vi "Test Get All Items.vi"(8 "error in (no error)":errorcluster, 11 "Result Model Result Recording Test in":refnum<class "Result Model Result Recording Test.lvclass">) -> (0 "error out":errorcluster, 3 "Result Model Result Recording Test out":refnum<class "Result Model Result Recording Test.lvclass">)   [LabVIEW 2020, in "Result Model Result Recording Test.lvclass"]
uses:
  Result Model Result Recording Test.lvclass
  Result Model Result Recording Test.lvclass/Result Model Result Recording Test.ctl
  Result Model/Result Model.lvclass
  Result/Type.ctl
  Result/Result.lvlib
  Result/Status.ctl
  Result/Result.ctl
  ae2c71b8-32bb-49d1-8500-0119bfec74ff.vi
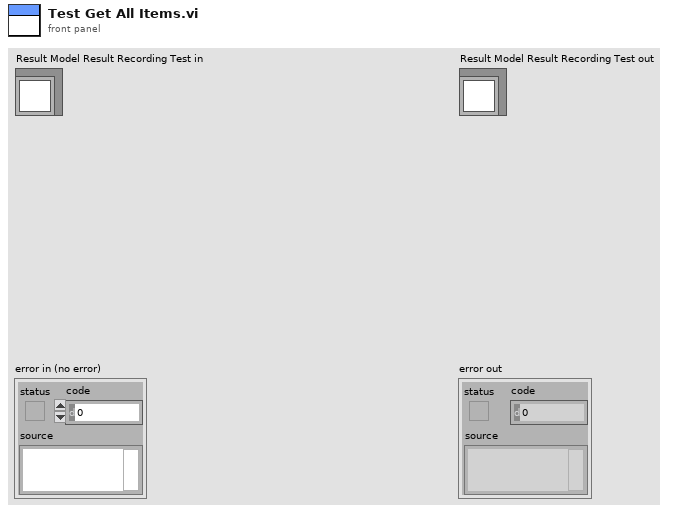
[diagram p1: front panel]
types:
  T1 = typedef "Result.lvlib/Result.ctl" = cluster{"Name":string, "Message":string, "Description":string, "Status":T2, "Result Type":T3, "Execution Time":dbl}
  T2 = typedef "Result.lvlib/Status.ctl" = enum16{"", "Passed", "Failed", "Error", "Skipped", "Setup Error", "Broken", "Teardown Error"}
  T3 = typedef "Result.lvlib/Type.ctl" = enum16{"Method", "Case", "Suite", "Pass", "Fail", "Skip", "Pass if", "Fail if", "Pass if Error", "Fail if Error", "Pass if Equal", "Fail if Equal"}
  T4 = cluster{"Left Cell String":string, "Child Text":string[], "Child Tag":string, "Item Indent":i32, "Child Only?":bool, "Glyph Index":i32}[]
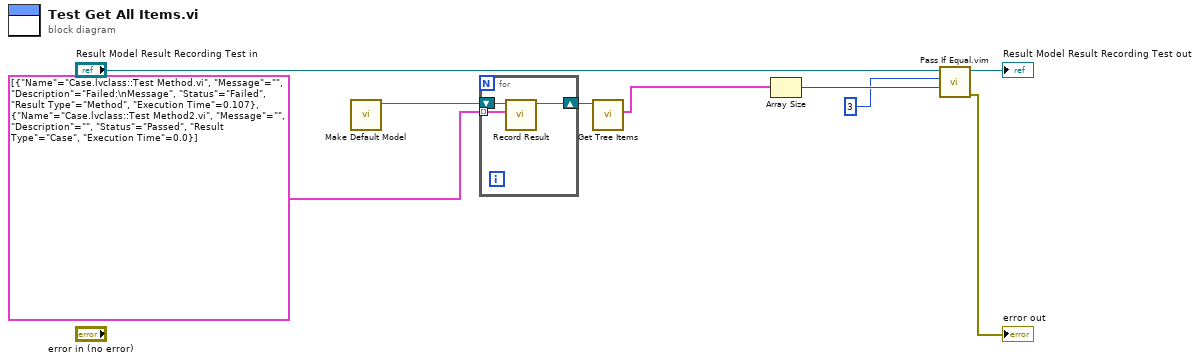
[diagram p0: block diagram]
diagram:
  n1 = call "Make Default Model.vi"() -> ("Result Model out"=w9:refnum<class "Result Model.lvclass">)  [unwired: 10 in, 1 out]
  n2 = for {
    tunnel: T1[] [{"Name"="Case.lvclass::Test Method.vi", "Message"="", "Description"="Failed:\nMessage", "Status"=enum."Failed", "Result Type"=enum."Method", "Execution Time"=0.107}, {"Name"="Case.lvclass::Test Method2.vi", "Message"="", "Description"="", "Status"=enum."Passed", "Result Type"=enum."Case", "Execution Time"=0.0}] ("Results") -> [w11] mode=indexing
    shift-right: [w10] -> w7
    shift-left: w9 -> [w12]
    n3 = call "Record Result.vi"("Results"=w11, "Result Model in"=w12) -> ("Result Model out"=w10:refnum<class "Result Model.lvclass">)  [unwired: 9 in]
  }
  n4 = call "Get Tree Items.vi"("Result Model In"=w7) -> ("Tree Items"=w6:T4)  [unwired: 9 in, 1 out]
  n5 = Array Size(array=w6) -> (size(s)=w2:i32)
  n6 = call "Pass If Equal.vim"("Actual"=w2, "Expected"=3 ("size(s)"), "LUnit Test Case In"="Result Model Result Recording Test in") -> ("error out"=→"error out":errorcluster, "LUnit Test Case Out"=→"Result Model Result Recording Test out":refnum<class "Result Model Result Recording Test.lvclass">)  [unwired: 7 in]
